vi "PAM Array Buffer Size.vi"() -> ()   [LabVIEW 2020, in "PAM Library.lvlib"]
uses:
  PAM Library.lvlib
panel:
  in  "PAM Array Buffer Size":i32
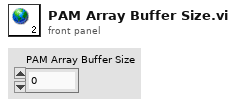
[diagram p1: front panel]
diagram:
